vi "DB_EscribeTablaPower.vi"(8 "error in (no error)":errorcluster, 9 "Power_cluster":T1, 10 "Equipo_Medicion":T2={"ID_EQUIPO"=0, "IP_EQUIPO"="", "NOMBRE_EQUIPO"="", "ESTADO_EQUIPO"="", "DESCRIPCION"="", "ID_MEDICION"=0, "ESTADO_MEDICION"="", "TIEMPO_MEDICION"="12-02-2019 18:41"}, 11 "db in":T3) -> (0 "error out":errorcluster, 3 "db out":T3)   [LabVIEW 2018]
uses:
  <vilib>/addons/database/Connection.llb/Conn ObjectReference.ctl
  Controls/Equipos_Medicion_cluster.ctl
  Controls/Power_cluster.ctl
  <vilib>/addons/database/Connection.llb/Conn Execute.vi
  <vilib>/addons/database/Recordset.llb/Rec Destroy - Connection.vi
  <vilib>/addons/database/NI_Database_API.lvlib
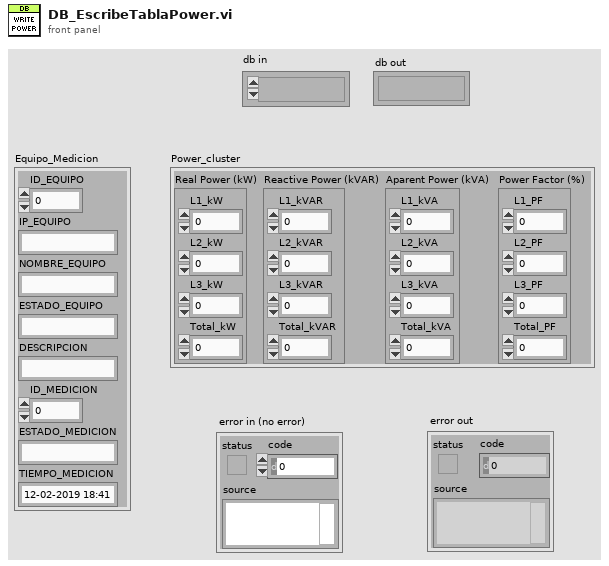
[diagram p1: front panel]
types:
  T1 = typedef "Power_cluster.ctl" = cluster{"Real Power (kW)":cluster{"L1_kW":sgl, "L2_kW":sgl, "L3_kW":sgl, "Total_kW":sgl}, "Reactive Power (kVAR)":cluster{"L1_kVAR":sgl, "L2_kVAR":sgl, "L3_kVAR":sgl, "Total_kVAR":sgl}, "Aparent Power (kVA)":cluster{"L1_kVA":sgl, "L2_kVA":sgl, "L3_kVA":sgl, "Total_kVA":sgl}, "Power Factor (%)":cluster{"L1_PF":sgl, "L2_PF":sgl, "L3_PF":sgl, "Total_PF":sgl}}
  T2 = typedef "Equipos_Medicion_cluster.ctl" = cluster{"ID_EQUIPO":i32, "IP_EQUIPO":string, "NOMBRE_EQUIPO":string, "ESTADO_EQUIPO":string, "DESCRIPCION":string, "ID_MEDICION":i32, "ESTADO_MEDICION":string, "TIEMPO_MEDICION":string}
  T3 = typedef "NI_Database_API.lvlib/Conn ObjectReference.ctl" = refnum<k1>
  T4 = cluster{"L1_kW":sgl, "L2_kW":sgl, "L3_kW":sgl, "Total_kW":sgl}
  T5 = cluster{"L1_kVAR":sgl, "L2_kVAR":sgl, "L3_kVAR":sgl, "Total_kVAR":sgl}
  T6 = cluster{"L1_kVA":sgl, "L2_kVA":sgl, "L3_kVA":sgl, "Total_kVA":sgl}
  T7 = cluster{"L1_PF":sgl, "L2_PF":sgl, "L3_PF":sgl, "Total_PF":sgl}
  T8 = typedef "NI_Database_API.lvlib/Rec ObjectReference.ctl" = refnum<k1>
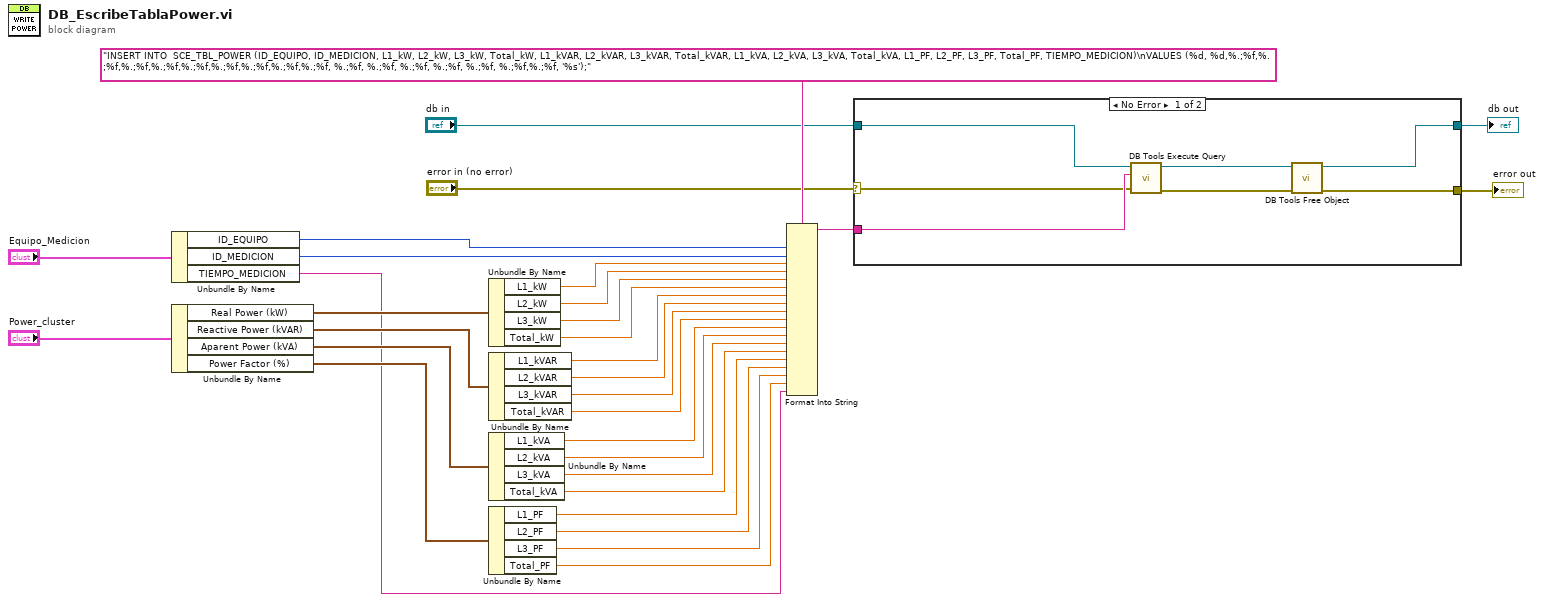
[diagram p0: block diagram]
diagram:
  n1 = Unbundle By Name("Equipo_Medicion") -> ("ID_EQUIPO"=w27:i32, "ID_MEDICION"=w26:i32, "TIEMPO_MEDICION"=w5:string)
  n2 = Unbundle By Name("Power_cluster") -> ("Real Power (kW)"=w19:T4, "Reactive Power (kVAR)"=w18:T5, "Aparent Power (kVA)"=w17:T6, "Power Factor (%)"=w16:T7)
  n3 = Unbundle By Name(w19) -> ("L1_kW"=w25:sgl, "L2_kW"=w24:sgl, "L3_kW"=w23:sgl, "Total_kW"=w11:sgl)
  n4 = Unbundle By Name(w18) -> ("L1_kVAR"=w22:sgl, "L2_kVAR"=w21:sgl, "L3_kVAR"=w20:sgl, "Total_kVAR"=w9:sgl)
  n5 = Unbundle By Name(w17) -> ("L1_kVA"=w10:sgl, "L2_kVA"=w15:sgl, "L3_kVA"=w14:sgl, "Total_kVA"=w8:sgl)
  n6 = Unbundle By Name(w16) -> ("L1_PF"=w7:sgl, "L2_PF"=w13:sgl, "L3_PF"=w12:sgl, "Total_PF"=w6:sgl)
  n7 = Format Into String(format string="INSERT INTO  SCE_TBL_POWER (ID_EQUIPO, ID_MEDICION, L1_kW, L2_kW, L3_kW, Total_kW, L1_kVAR, L2_kVAR, L3_kVAR, Total_kVAR, L1_kVA, L2_kVA, L3_kVA, Total_kVA, L1_PF, L2_PF, L3_PF, Total_PF, TIEMPO_MEDICION)\nVALUES (%d, %d,%.;%f,%.;%f,%.;%f,%.;%f,%.;%f,%.;%f,%.;%f,%.;%f,%.;%f, %.;%f, %.;%f, %.;%f, %.;%f, %.;%f, %.;%f,%.;%f, '%s');" ("SQL"), w27, w26, w25, w24, w23, w11, w22, w21, w20, w9, w10, w15, w14, w8, w7, w13, w12, w6, w5) -> (resulting string=w31:string)  [unwired: 2 in, 1 out]
  n8 = case shown="No Error" "error in (no error)" {
    selector: "error in (no error)" -> [w36 w40]
    tunnel: w31 -> [w37 _]
    tunnel: [w34 w40] -> w29
    tunnel: "db in" -> [w35 w39]
    tunnel: [w32 w39] -> w3
    frame No Error {
      n9 = call-poly <vilib>:"DB Tools Execute Query.vi"("error in (no error)"=w36, "SQL query"=w37, "connection reference"=w35) -> ("error out"=w38:errorcluster, "recordset reference"=w33:T8)  [unwired: 5 in]
      n10 = call-poly <vilib>:"DB Tools Free Object.vi"("error in (no error)"=w38, "recordset reference"=w33) -> ("error out"=w34:errorcluster, "connection reference"=w32:T3)  [unwired: 8 in]
    }
    frame Error {
    }
  }
  "error out" <- w29
  "db out" <- w3
